vi "UNIX Timestamp.vi"() -> (3 "UNIX Time Stamp":timestamp format="%<%x %.3X>T")   [LabVIEW 2020, in "InfluxDB v2 Client.lvlib"]
doc: "This VI converts from the LabVIEW based time (epoch Jan. 1, 1904) to UNIX time (epoch Jan. 1, 1970)."
uses:
  InfluxDB v2 Client.lvlib
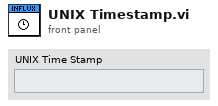
[diagram p1: front panel]
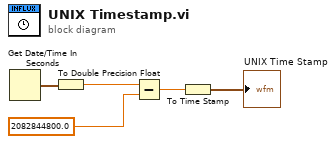
[diagram p0: block diagram]
diagram:
  n1 = Get Date/Time In Seconds() -> (seconds since 1Jan1904=w2:timestamp)
  n2 = To Double Precision Float(number=w2) -> (double precision float=w1:dbl)
  n3 = Subtract(x=w1, y=2082844800.0) -> (x-y=w4:dbl)
  n4 = To Time Stamp(1:w4) -> (0:→"UNIX Time Stamp":timestamp)
